vi "Result Parser.vi"(11 "operation":u32) -> (2 "address":u8=97 format="%.0x", 3 "data":u8=97 format="%.0x", 5 "busy flag":bool)   [LabVIEW 2017, in "HD44780 Common.lvlib"]
uses:
  HD44780 Common.lvlib
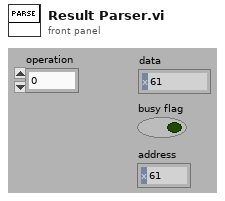
[diagram p1: front panel]
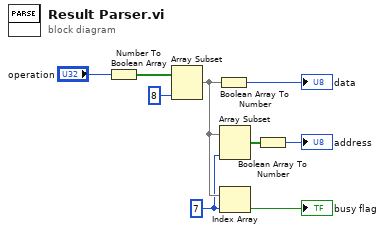
[diagram p0: block diagram]
diagram:
  w7 = 7 ("index")
  n1 = Number To Boolean Array(number="operation") -> (Boolean array=w6:bool[])
  n2 = Array Subset(array=w6, length=8) -> (w8:bool[])  [unwired: 1 in]
  n3 = Boolean Array To Number(Boolean array=w8) -> (number=→"data":u8)
  n4 = Array Subset(array=w8, length=w7) -> (w3:bool[])  [unwired: 1 in]
  n5 = Index Array(array=w8, index=w7) -> (element=→"busy flag":bool)
  n6 = Boolean Array To Number(Boolean array=w3) -> (number=→"address":u8)
